vi "Init HTTP Service.vi"(8 "error in (no error)":errorcluster, 11 "Vecto in":refnum<class "Vecto.lvclass">) -> (0 "error out":errorcluster, 3 "Vecto out":refnum<class "Vecto.lvclass">)   [LabVIEW 2020, in "Vecto.lvlib" / "Vecto.lvclass"]
uses:
  Vecto.lvclass
  Vecto.lvclass/Vecto.ctl
  Service Container/Service Container.lvclass
  C:/Program Files (x86)/National Instruments/LabVIEW 2020/vi.lib/IlluminatedG/IG HTTP Server/HTTP Server/Service/Service.lvclass
  HTTPServerService/HTTPServerService.lvclass
  C:/dev/lv20CE/lv-vecto/Vecto/Service/Service.lvclass
  <vilib>/IlluminatedG/IG HTTP Server/HTTP Server/Server/Server.lvclass
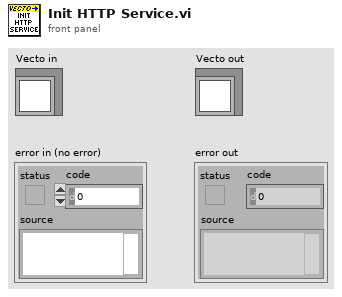
[diagram p1: front panel]
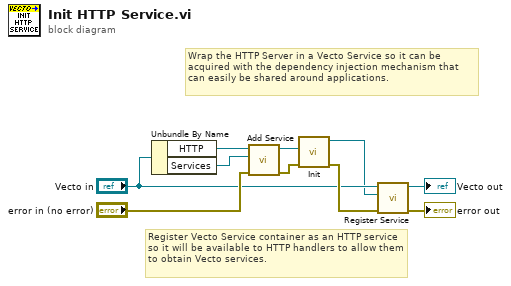
[diagram p0: block diagram]
diagram:
  # "Register Vecto Service container as an HTTP service so it will be available to HTTP handlers to allow them to obtain Vecto services."
  # "Wrap the HTTP Server in a Vecto Service so it can be acquired with the dependency injection mechanism that can easily be shared around applications."
  n1 = Unbundle By Name("Vecto in") -> ("HTTP"=w4:refnum<class "Server.lvclass">, "Services"=w3:refnum<class "Service Container.lvclass">)
  n2 = call <vilib>:"Add Service.vi"("error in (no error)"="error in (no error)", "Service"=w3, "Server in"=w4) -> ("error out"=w1:errorcluster, "Server out"=w2:refnum<class "Server.lvclass">)  [unwired: 7 in]
  n3 = call "Init.vi"("error in (no error)"=w1, "HTTP Server"=w2) -> ("error out"=w10:errorcluster, "HTTPServerService out"=w7:refnum<class "HTTPServerService.lvclass">)  [unwired: 8 in]
  n4 = call "Register Service.vi"("error in (no error)"=w10, "Service"=w7, "Vecto in"="Vecto in") -> ("error out"=→"error out":errorcluster, "Vecto out"=→"Vecto out":refnum<class "Vecto.lvclass">)  [unwired: 7 in]
